vi "Z6_Beamline.constructor.vi"(0 "name":string, 2 "data in":string, 5 "error in":errorcluster) -> (14 "i ref out":refnum<vi>, 16 "data out":string, 19 "error out":errorcluster)   [LabVIEW 2014, in "Z6_Beamline.lvlib"]
doc: "This class is forseen to inspect the PHELIX beamline and to select the mode. Additional several settings can be chosen.\n\nThis class is part of the PHELIX user layer.\n\nauthor: Stefan Götte, GSI\n\nLicense Agreement for this software:\n\nCopyright (C)\nGesellschaft für Schwerionenforschung, GSI\nPlanckstr. 1\n64291 Darmstadt\nGermany\n\nContact: D.Beck@gsi.de \n\nThis program is free software; you can redistribute it and/or modify it under the terms of the \nGNU General Public License as published by the Free Software Foundation; either version 2 of \nthe license, or (at your option) any later version.\n\nThis program is distributed in the hope that it will be useful, but WITHOUT ANY WARRANTY; \nwithout even the implied warranty of MERCHANTABILITY or FITNESS FOR A PARTICULAR PURPOSE. See the GNU General License for more details (http://www.gnu.org).\n\nGesellschaft für Schwerionenforschung, GSI\nPlanckstr. 1, 64291 Darmstadt, Germany\nFor all questions and ideas contact: M.Richter@gsi.de, H.Brand@gsi.de or D.Beck@gsi.de.\nLast update: 16-JUN-2004"
uses:
  Z6_Beamline.lvlib
  CSCore/CSSystem/CSSystemLib/CSSystemLib.lvlib
  PH_BL-Master/PH_BL-Master.lvlib
  PH_Class/PH_Class.lvlib
  CSCore/CSObj/CSObj.lvlib
  PH_Common/PH_Common.lvlib
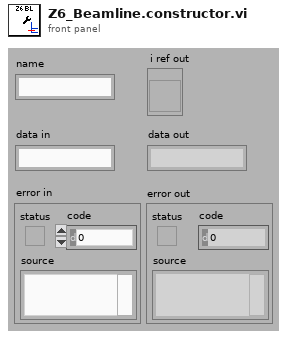
[diagram p1: front panel]
types:
  T1 = enum16{"SetAttribute", "GetAttribute", "CreateAttribute", "DestroyAttribute", "DestroyAllAtributes"}
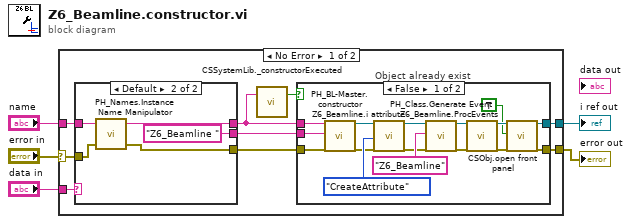
[diagram p0: block diagram]
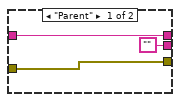
[diagram p2: hidden frame]
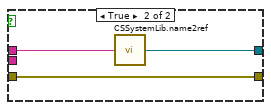
[diagram p3: hidden frame]
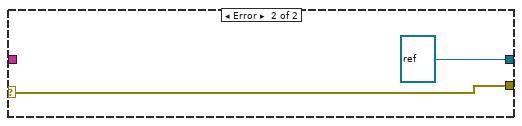
[diagram p4: hidden frame]
diagram:
  n1 = case shown="No Error" "error in" {
    selector: "error in" -> [w10 w43]
    tunnel: "name" -> [w11 _]
    tunnel: [w13 w43] -> w4
    tunnel: [w12 refnum<vi> refnum ("i ref out")] -> w5
    tunnel: "data in" -> [w6 _]
    frame No Error {
      n2 = case shown="Default" w6 {
        tunnel: w11 -> [w16 w22]
        tunnel: w10 -> [w17 w21]
        tunnel: [w17 w20] -> w9
        tunnel: [w16 w19] -> w8
        tunnel: ["" "Z6_Beamline "] -> w7
        frame "Parent" {
        }
        frame Default {
          n3 = call "PH_Names.Instance Name Manipulator.vi"("error in (no error)"=w21, "name in"=w22) -> ("error out"=w20:errorcluster, "name out"=w19:string)  [unwired: 1 in, 1 out]
        }
      }
      n4 = call "CSSystemLib._constructorExecuted.vi"("name"=w8) -> ("constructor executed?"=w14:bool)  [unwired: 18 in]
      n5 = case "Object already exist" shown="False" w14 {
        tunnel: w8 -> [w37 w41]
        tunnel: [w25 w40] -> w13
        tunnel: w9 -> [w29 w40]
        tunnel: [w26 w39] -> w12
        tunnel: w7 -> [w23 _]
        frame False {
          n6 = call "PH_BL-Master.constructor.vi"("name"=w37, "data in"=w23, "error in"=w29) -> ("i ref out"=w35:refnum<vi>, "error out"=w34:errorcluster)  [unwired: 14 in, 1 out]
          n7 = call "Z6_Beamline.i attribute.vi"("VI Refnum"=w35, "Action"=T1."CreateAttribute", "error in (no error)"=w34) -> ("VI Refnum out"=w33:refnum<vi>, "error out"=w31:errorcluster)  [unwired: 14 in, 1 out]
          n8 = call "PH_Class.Generate Event.vi"("i ref in"=w33, "Class"="Z6_Beamline", "error in (no error)"=w31) -> ("i ref out"=w32:refnum<vi>, "error out"=w30:errorcluster)  [unwired: 15 in]
          n9 = call "Z6_Beamline.ProcEvents.vi"("i ref in"=w32, "error in (no error)"=w30) -> ("i ref out"=w27:refnum<vi>, "error out"=w28:errorcluster)  [unwired: 16 in]
          n10 = call "CSObj.open front panel.vi"("i ref in"=w27, "frontPanelOpen"=TRUE, "error in (no error)"=w28) -> ("i ref out"=w26:refnum<vi>, "error out"=w25:errorcluster)  [unwired: 15 in]
        }
        frame True {
          n11 = call "CSSystemLib.name2ref.vi"("name"=w41) -> ("obj refnum"=w39:refnum<vi>)
        }
      }
    }
    frame Error {
    }
  }
  "i ref out" <- w5
  "error out" <- w4
